vi "Delete Compilation Notes.vi"(8 "error in (no error)":errorcluster, 10 "note key":string, 11 "functionbase in":refnum<class "functionbase.lvclass">) -> (0 "error out":errorcluster, 3 "functionbase out":refnum<class "functionbase.lvclass">)   [LabVIEW 2019, in "LSL.lvlib" / "functionbase.lvclass"]
uses:
  functionbase.lvclass
  functionbase.lvclass/functionbase.ctl
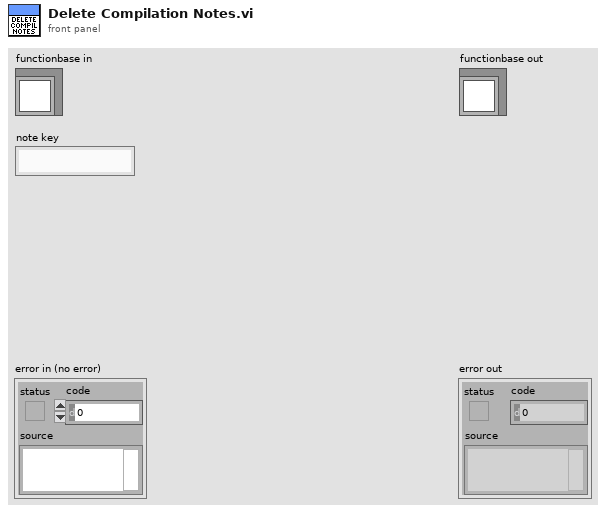
[diagram p1: front panel]
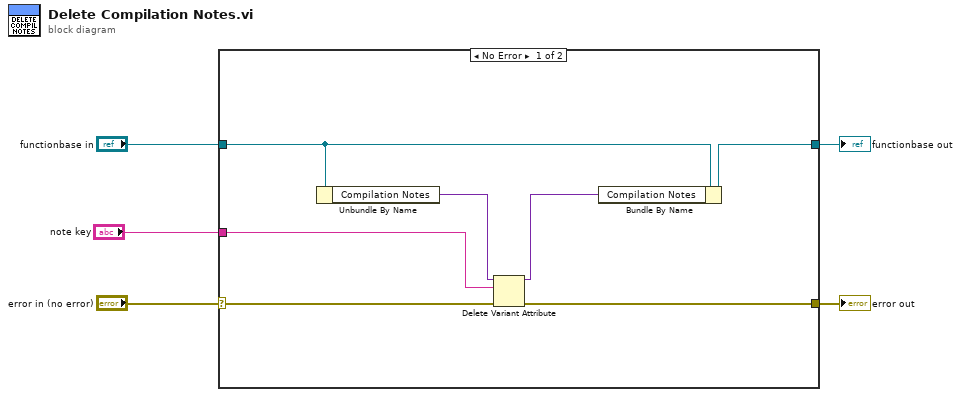
[diagram p0: block diagram]
diagram:
  n1 = case shown="No Error" "error in (no error)" {
    selector: "error in (no error)" -> [w12 w14]
    tunnel: [w11 w14] -> w4
    tunnel: [w8 w13] -> w2
    tunnel: "functionbase in" -> [w9 w13]
    tunnel: "note key" -> [w6 _]
    frame No Error {
      n2 = Unbundle By Name(w9) -> ("Compilation Notes"=w7:variant)
      n3 = Delete Variant Attribute(4:w12, 6:w6, 7:w7) -> (0:w11:errorcluster, 3:w10:variant)  [unwired: 1 out]
      n4 = Bundle By Name(cluster=w9, "Compilation Notes"=w10) -> (w8:refnum<class "functionbase.lvclass">)
    }
    frame Error {
    }
  }
  "error out" <- w4
  "functionbase out" <- w2
